vi "FT10_Calibration Calculate Gain.vi"(10 "Target":dbl[](array[numeric]), 11 "RMS Value":dbl[](array[numeric])) -> (1 "R-square":dbl, 2 "Intercept":dbl, 3 "Gain":dbl)   [LabVIEW 2015]
uses:
  <vilib>/Analysis/NI_AALPro.lvlib
panel:
  out "XY Graph":cluster{"Y":dbl[], "X":dbl[]}[](graph)
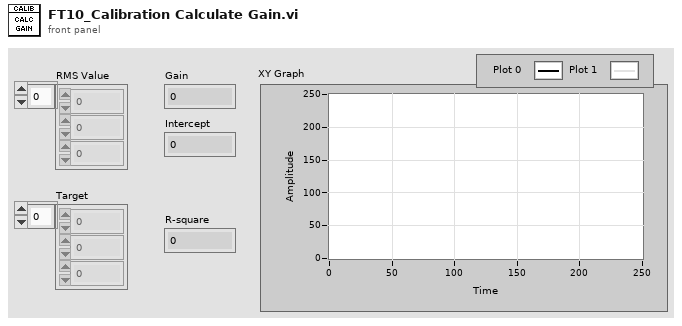
[diagram p1: front panel]
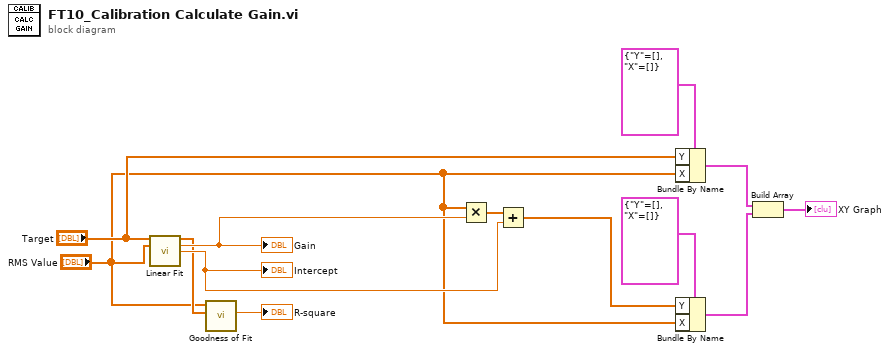
[diagram p0: block diagram]
diagram:
  n1 = call <vilib>:"Linear Fit.vi"("Y"="Target", "X"="RMS Value") -> ("Best Linear Fit"=w4:dbl[], "slope"=w10:dbl, "intercept"=w9:dbl)  [unwired: 9 in, 2 out]
  "Gain" <- w10
  "Intercept" <- w9
  n2 = call <vilib>:"Goodness of Fit.vi"("Best Fit"=w4, "Y"="RMS Value") -> ("R-square"=→"R-square":dbl)  [unwired: 6 in, 3 out]
  n3 = Multiply(x="RMS Value", y=w10) -> (x*y=w8:dbl[])
  n4 = Add(x=w8, y=w9) -> (x+y=w6:dbl[])
  n5 = Bundle By Name(cluster=cluster{"Y":dbl[], "X":dbl[]} {"Y"=[], "X"=[]} ("output cluster"), "Y"="Target", "X"="RMS Value") -> (w12:cluster{"Y":dbl[], "X":dbl[]})
  n6 = Bundle By Name(cluster=cluster{"Y":dbl[], "X":dbl[]} {"Y"=[], "X"=[]} ("output cluster"), "Y"=w6, "X"="RMS Value") -> (w5:cluster{"Y":dbl[], "X":dbl[]})
  n7 = Build Array(w12, w5) -> (→"XY Graph":cluster{"Y":dbl[], "X":dbl[]}[])
